vi "Set Moter Speed.vi"(2 "Buttons":T2, 3 "Axes":T1) -> (0 "right":dbl, 1 "left":dbl)   [LabVIEW 2011]
uses:
  <vilib>/Rock Robotics/WPI/Joystick/WPI_JoystickButtonState.ctl
  Robot Global Data.vi
panel:
  in  "Angle Tolerance":dbl=1.0
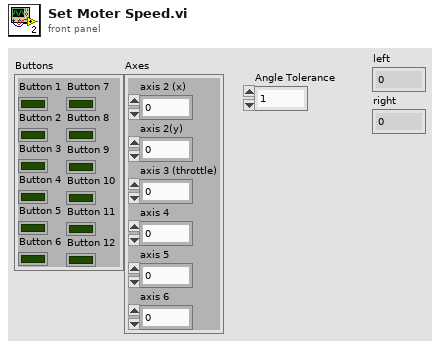
[diagram p1: front panel]
types:
  T1 = cluster{"axis 2 (x)":dbl, "axis 2(y)":dbl, "axis 3 (throttle)":dbl, "axis 4":dbl, "axis 5":dbl, "axis 6":dbl}
  T2 = typedef "WPI_JoystickButtonState.ctl" = cluster{"Button 1":bool, "Button 2":bool, "Button 3":bool, "Button 4":bool, "Button 5":bool, "Button 6":bool, "Button 7":bool, "Button 8":bool, "Button 9":bool, "Button 10":bool, "Button 11":bool, "Button 12":bool}
  T3 = typedef "WPI_GyroDevRef.ctl" = cluster{"DevStatus":errorcluster, "Analog Module":T4, "Analog Channel":T5, "Offset":dbl, "Gain (VoltsPerDegree/Second)":dbl}
  T4 = typedef "FPGA_TypedefAnalogModule.ctl" = enum16{"Analog Module 1", "Analog Module 2"}
  T5 = typedef "FPGA_AIChannel.ctl" = enum8{"AI 1", "AI 2", "AI 3", "AI 4", "AI 5", "AI 6", "AI 7", "AI 8", "Invalid"}
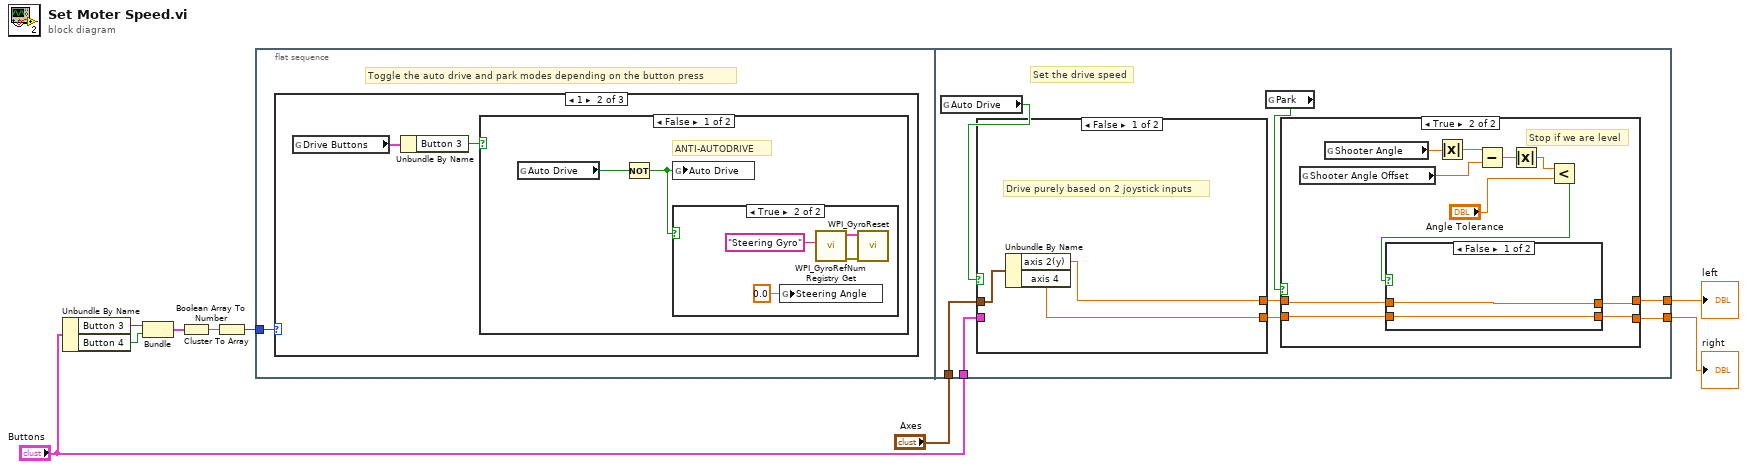
[diagram p0: block diagram]
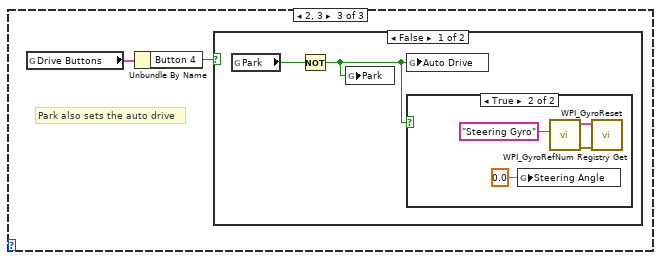
[diagram p5: hidden frame]
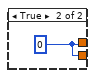
[diagram p9: hidden frame]
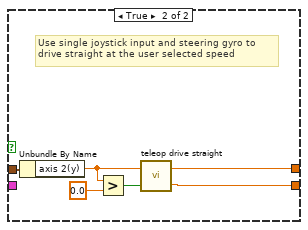
[diagram p10: hidden frame]
diagram:
  n1 = Unbundle By Name("Buttons") -> ("Button 3"=w5:bool, "Button 4"=w4:bool)
  n2 = Bundle("Button 3"=w5, "Button 4"=w4) -> (w3:cluster{"Button 3":bool, "Button 4":bool})  [unwired: 1 in]
  n3 = Cluster To Array(cluster=w3) -> (array=w2:bool[])
  n4 = Boolean Array To Number(Boolean array=w2) -> (number=w1:u32)
  n5 = flat-sequence {
    tunnel: w1 -> [w10]
    tunnel: "Axes" -> [w33]
    tunnel: "Buttons" -> [w32]
    tunnel: [w27] -> w7
    tunnel: [w28] -> w6
    frame #0 {
      # "Toggle the auto drive and park modes depending on the button press"
      n6 = case shown="1" w10 {
        frame 0, Default {
        }
        frame 1 {
          n7 = global read "Robot Global Data.vi" "Drive Buttons"() -> (w12:T2)
          n8 = Unbundle By Name(w12) -> ("Button 3"=w11:bool)
          n9 = case shown="False" w11 {
            frame False {
              # "ANTI-AUTODRIVE"
              n10 = global read "Robot Global Data.vi" "Auto Drive"() -> (w14:bool)
              n11 = Not(x=w14) -> (.not. x?=w13:bool)
              n12 = global write "Robot Global Data.vi" "Auto Drive"(w13) -> ()
              n13 = case shown="True" w13 {
                frame False {
                }
                frame True {
                  n14 = global write "Robot Global Data.vi" "Steering Angle"(0.0 ("Steering Angle")) -> ()
                  n15 = call <vilib>:"WPI_GyroRefNum Registry Get.vi"("refnum name"="Steering Gyro") -> ("error out"=w17:errorcluster, "GyroDevRef"=w16:T3)  [unwired: 9 in]
                  n16 = call <vilib>:"WPI_GyroReset.vi"("error in (no error)"=w17, "GyroDevRef"=w16) -> ()  [unwired: 8 in, 2 out]
                }
              }
            }
            frame True {
            }
          }
        }
        frame 2, 3 {
          # "Park also sets the auto drive"
          n17 = global read "Robot Global Data.vi" "Drive Buttons"() -> (w20:T2)
          n18 = Unbundle By Name(w20) -> ("Button 4"=w19:bool)
          n19 = case shown="False" w19 {
            frame False {
              n20 = global read "Robot Global Data.vi" "Park"() -> (w22:bool)
              n21 = Not(x=w22) -> (.not. x?=w21:bool)
              n22 = global write "Robot Global Data.vi" "Park"(w21) -> ()
              n23 = global write "Robot Global Data.vi" "Auto Drive"(w21) -> ()
              n24 = case shown="True" w21 {
                frame False {
                }
                frame True {
                  n25 = global write "Robot Global Data.vi" "Steering Angle"(0.0 ("Steering Angle")) -> ()
                  n26 = call <vilib>:"WPI_GyroRefNum Registry Get.vi"("refnum name"="Steering Gyro") -> ("error out"=w25:errorcluster, "GyroDevRef"=w24:T3)  [unwired: 9 in]
                  n27 = call <vilib>:"WPI_GyroReset.vi"("error in (no error)"=w25, "GyroDevRef"=w24) -> ()  [unwired: 8 in, 2 out]
                }
              }
            }
            frame True {
            }
          }
        }
      }
    }
    frame #1 {
      # "Set the drive speed"
      n28 = global read "Robot Global Data.vi" "Auto Drive"() -> (w34:bool)
      n29 = case shown="False" w34 {
        tunnel: w33 -> [w53 w59]
        tunnel: w32 -> [_ _]
        tunnel: [w52 w58] -> w30
        tunnel: [w51 w57] -> w29
        frame False {
          # "Drive purely based on 2 joystick inputs"
          n30 = Unbundle By Name(w53) -> ("axis 2(y)"=w52:dbl, "axis 4"=w51:dbl)
        }
        frame True {
          # "Use single joystick input and steering gyro to \ndrive straight at the user selected speed"
          n31 = Unbundle By Name(w59) -> ("axis 2(y)"=w56:dbl)
          n32 = Greater?(x=w56, y=0.0) -> (0:w54:bool)
          n33 = call "teleop drive straight.vi"("Reverse"=w54, "Speed"=w56) -> ("right"=w57:dbl, "left"=w58:dbl)
        }
      }
      n34 = global read "Robot Global Data.vi" "Park"() -> (w31:bool)
      n35 = case shown="True" w31 {
        tunnel: w30 -> [w35 w44]
        tunnel: [w36 w41] -> w28
        tunnel: w29 -> [w36 w43]
        tunnel: [w35 w42] -> w27
        frame False {
        }
        frame True {
          # "Stop if we are level"
          n36 = global read "Robot Global Data.vi" "Shooter Angle Offset"() -> (w39:dbl)
          n37 = global read "Robot Global Data.vi" "Shooter Angle"() -> (w47:dbl)
          n38 = Absolute Value(x=w47) -> (abs(x)=w40:dbl)
          n39 = Subtract(x=w40, y=w39) -> (x-y=w38:dbl)
          n40 = Absolute Value(x=w38) -> (abs(x)=w37:dbl)
          n41 = Less?(x=w37, y="Angle Tolerance") -> (x < y?=w45:bool)
          n42 = case shown="False" w45 {
            tunnel: w44 -> [w48 _]
            tunnel: [w49 w50] -> w41
            tunnel: w43 -> [w49 _]
            tunnel: [w48 w50] -> w42
            frame False {
            }
            frame True {
              w50 = 0
            }
          }
        }
      }
    }
  }
  "left" <- w7
  "right" <- w6
